vi "Object recognition.vi"() -> ()   [LabVIEW 2018]
uses:
  <vilib>/userdefined/High Color/IMAQdx.ctl
  Underlying VI's/Webcam FGV Low level ver/State control.ctl
panel:
  out "Error out":errorcluster
  in  "stop":bool
  out "Image":T1(plugin-control)
  out "Object Center Coordinates":cluster{"x":sgl, "y":sgl}
  out "Object detection cluster":T2
  in  "Mode":enum16{"Ball", "Soap", "Gel", "Pipe", "None"}(ring)
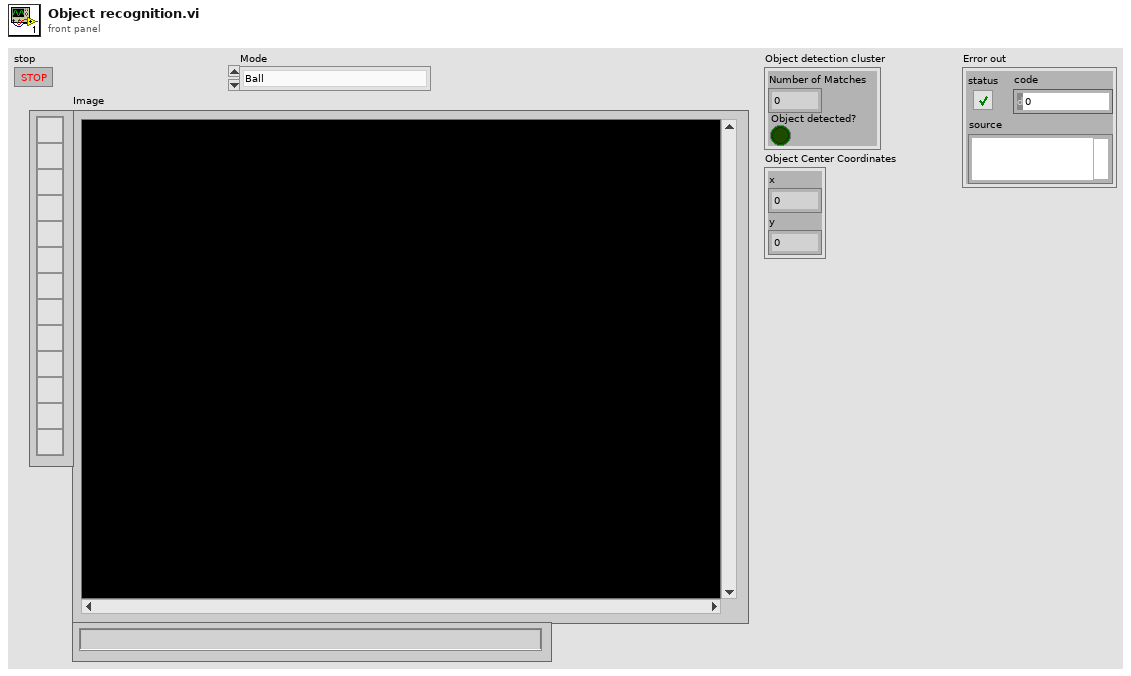
[diagram p1: front panel]
types:
  T1 = typedef "IMAQ Image.ctl" = refnum<image>
  T2 = cluster{"Number of Matches":i32, "Object detected?":bool}
  T3 = typedef "State control.ctl" = enum16{"Initialise", "Start camera", "Continuous Acquisition ", "Stop camera", "Dispose all"}
  T4 = typedef "IMAQdx.ctl" = refnum<k21>
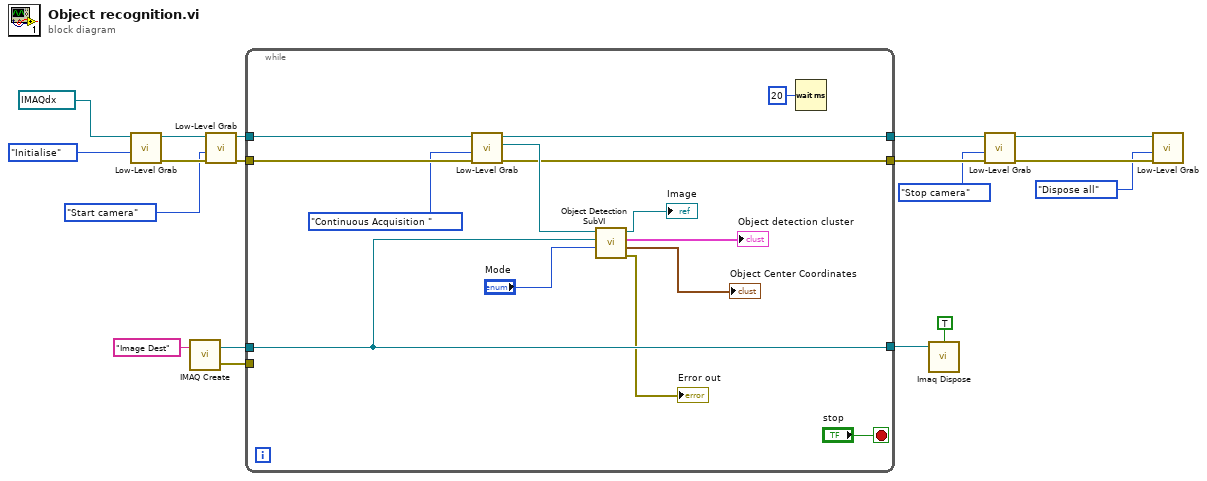
[diagram p0: block diagram]
diagram:
  n1 = call "Low-Level Grab.vi"("States"=State_control."Initialise", "Session In"=T4 "cam0") -> ("error out"=w17:errorcluster, "Session Out"=w18:T4)  [unwired: 7 in, 1 out]
  n2 = call "IMAQ Create"("Image Name"="Image Dest") -> ("New Image"=w5:T1, "error out"=w2:errorcluster)  [unwired: 4 in]
  n3 = call "Low-Level Grab.vi"("error in (no error)"=w17, "States"=State_control."Start camera", "Session In"=w18) -> ("error out"=w13:errorcluster, "Session Out"=w12:T4)  [unwired: 6 in, 1 out]
  n4 = while {
    tunnel: w13 -> [w31]
    tunnel: w12 -> [w32]
    tunnel: [w28] -> w11
    tunnel: [w27] -> w10
    tunnel: w5 -> [w20]
    tunnel: [w20] -> w3
    tunnel: w2 -> [_]
    stop <- "stop" stop-if-true
    n5 = call "Low-Level Grab.vi"("error in (no error)"=w31, "States"=State_control."Continuous Acquisition ", "Session In"=w32) -> ("error out"=w27:errorcluster, "Image Out"=w29:T1, "Session Out"=w28:T4)  [unwired: 6 in]
    n6 = call "Object Detection SubVI.vi"("Mode"="Mode", "Image Dest"=w20, "Image in"=w29) -> ("Error out"=→"Error out":errorcluster, "Object Center Coordinates"=→"Object Center Coordinates":cluster{"x":sgl, "y":sgl}, "Object detection cluster"=→"Object detection cluster":T2, "Image Out"=→"Image":T1)  [unwired: 1 in]
    n7 = Wait (ms)(milliseconds to wait=u32 20) -> ()  [unwired: 1 out]
  }
  n8 = call "Imaq Dispose"("All Images? (No)"=TRUE, "Image"=w3) -> ()  [unwired: 4 in, 1 out]
  n9 = call "Low-Level Grab.vi"("error in (no error)"=w10, "States"=State_control."Stop camera", "Session In"=w11) -> ("error out"=w8:errorcluster, "Session Out"=w9:T4)  [unwired: 6 in, 1 out]
  n10 = call "Low-Level Grab.vi"("error in (no error)"=w8, "States"=State_control."Dispose all", "Session In"=w9) -> ()  [unwired: 6 in, 3 out]
